vi "PS_Main_two_polarimeters.vi"() -> ()   [LabVIEW 2011]
uses:
  PS_Global.vi
  <vilib>/express/express arith-compare/Formula/XNode/ExpressFormulaBlockNode.xnode
panel:
  out "Offsets at Both Wave Plate Settings":dbl[][](array[numeric])
  in  "Polarimeter Angles":dbl[](array[numeric])
  out "Running Std":dbl[](array[numeric]) format="%#.2g%"
  out "Running Average":dbl[](array[numeric]) format="%#.1f%"
  out "Next Pol Value":dbl[](array[numeric])
  out "Polarization Graph":dynamicdata(graph)
  out "Offset: Laser off":dbl[](array[numeric])
  out "Offset: Laser on":dbl[](array[numeric])
  out "Corrected Lo":dbl[](array[numeric])
  out "Corrected Hi":dbl[](array[numeric])
  out "Optical Polarization":dbl[](array[numeric]) format="%#.1f%"
  out "Nuclear Polarization":dbl[](array[numeric]) format="%#.1f%"
  out "Std Lo":dbl[](array[numeric]) format="%.4f"
  out "Std Hi":dbl[](array[numeric]) format="%.4f"
  out "Mean Lo":dbl[](array[numeric]) format="%.4f"
  out "Mean Hi":dbl[](array[numeric]) format="%.4f"
  in  "# in avg":i32=1000
  in  "Init Running Avg":bool
  out "Counter":i32=1000
  out "Numbers to Avg":dbl[](array[numeric])
  in  "New Discharge ON":bool
  in  "Pressure Calib":dbl=0.553
  out "LCR V Min":dbl
  out "LCR Min V":dbl
  out "LCR Max V":dbl
  out "LCR Calibration Plot":cluster{"Y":dbl[], "Y":dbl[]}[](graph)
  in  "Calibrate LCR":bool
  in  "Discharge Voltage":dbl=10.3
  in  "Cell Pressure":dbl
  in  "stop":bool
  out "Heartbeat":string
  in  "Set All Offsets":bool
  in  "Run Polarimeter?":bool=TRUE
  out "Laser Global":bool
  in  "C8 Line?":bool caption="Laser State"
  out "Status":string
  out "Laser Peaks":cluster{dbl[], dbl[]}[](graph)
  out "Laser Peak Voltage Set":dbl format="%#_g V"
  in  "Run Laser Peak Find":bool
  in  "Lower Voltge Limit":dbl=1.2
  in  "Upper Voltage Limit":dbl=4.0
  in  "CP In?":bool
  in  "Comment Box":string
  in  "Insert Comment":bool
  in  "Plasma On Length":dbl=0.2
  out "Plasma On":dbl
  out "Plasma State":bool caption="Plasma Ball Status"
  out "Shutter Closed":dbl format="%.0f sec"
  in  "Shutter Set":bool=TRUE
  out "Shutter State":bool=TRUE caption="Shutter Status"
  out "Discharge State":bool caption="Discharge Status"
  in  "Discharge Set":bool
  out "Plasma On":timestamp
  out "Shutter Time":timestamp
  out "log":refnum<file>
  out "VI Running":bool
  out "Off Time":timestamp
  out "On Time":timestamp
  out "Decay Running":bool caption="Status"
  out "Start Time":timestamp
  out "Duration":dbl
  in  "Discharge Interval":dbl=30.0
  in  "Discharge Length":dbl=5.0
  in  "Run Decay":bool
  out "Messages":string
  in  "Laser State Set":bool caption="Laser State"
  in  "Get Signal Offset":bool
  in  "High Signal Extend":i32=280
  out "Signals":dynamicdata(graph) caption="Section"
  in  "High Signal Start":i32=400 caption="Begin Sample"
  in  "Low Signal Start":i32=120 caption="Begin Sample"
  in  "Number of Samples":i32=800
  in  "Sample Rate (Hz)":dbl=4000.0
  # "Set Laser State"
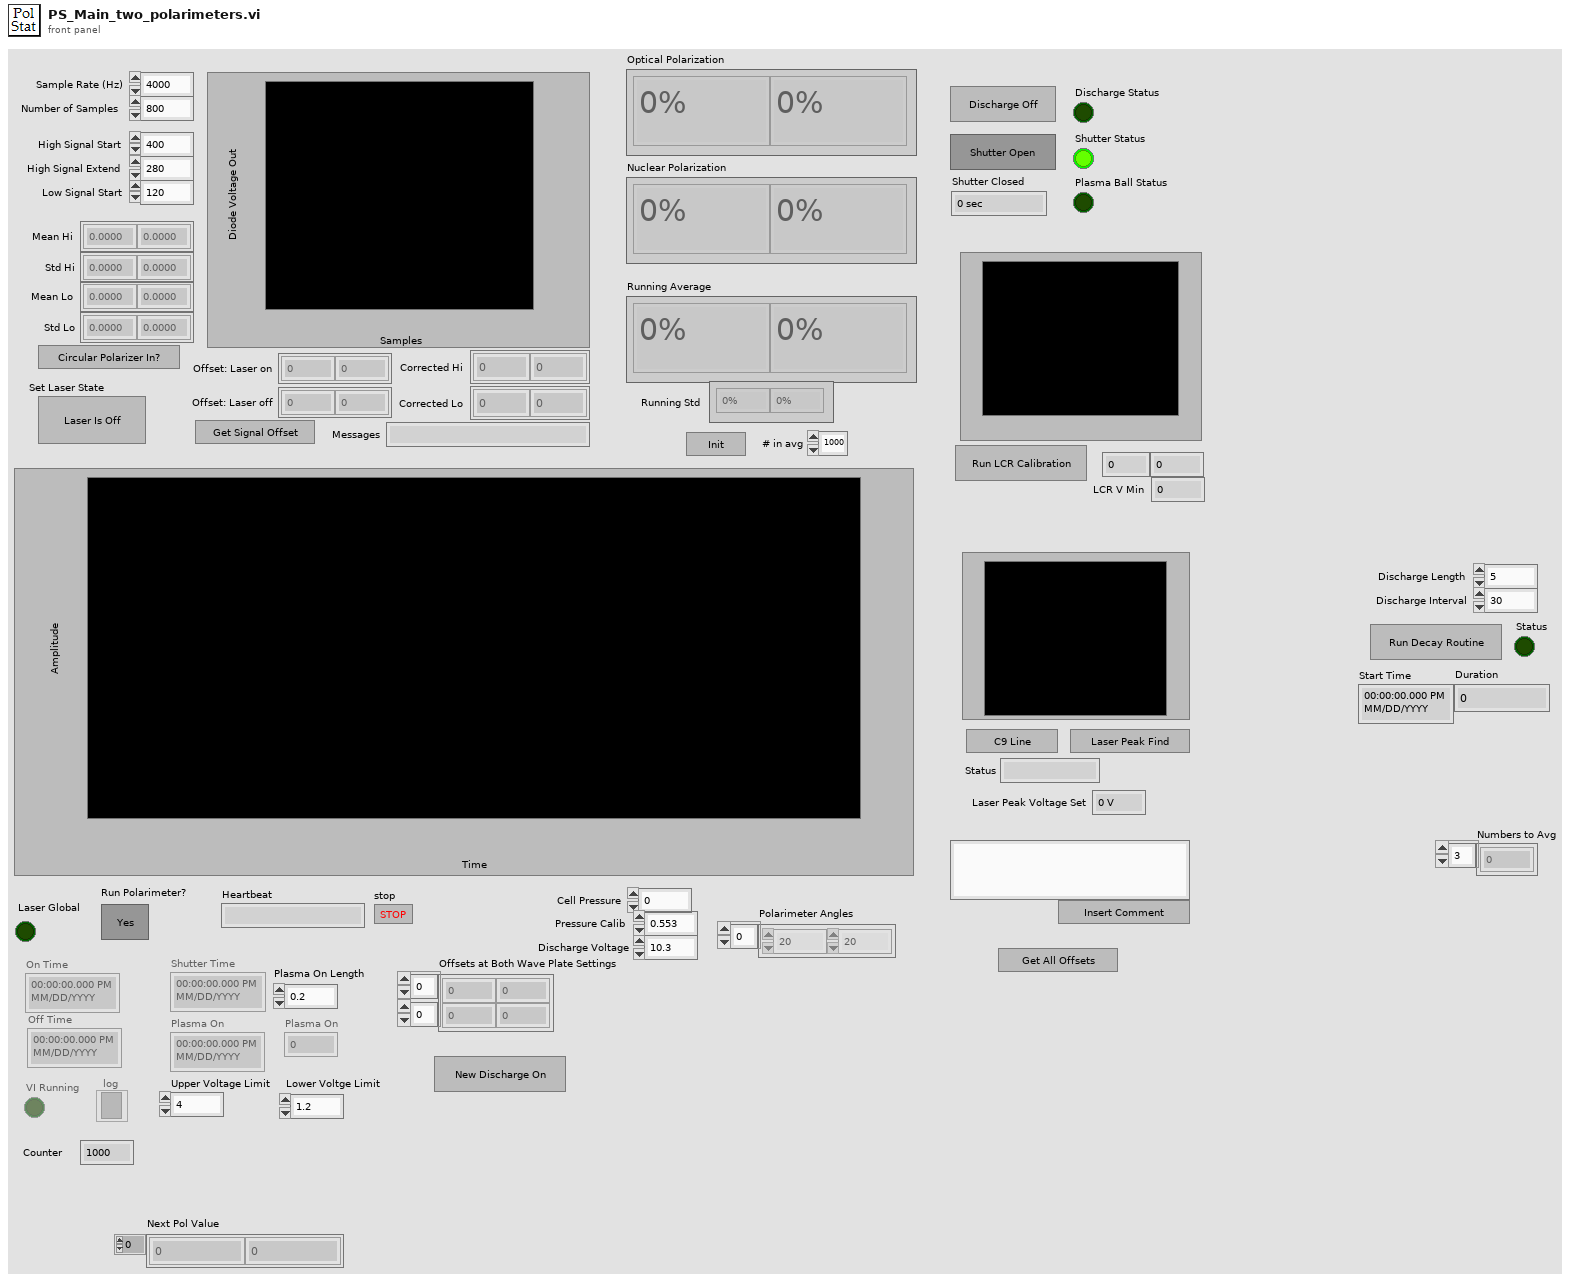
[diagram p1: front panel]
types:
  T1 = enum16{"open", "replace", "create", "open or create", "replace or create", "replace or create with confirmation"}
  T2 = enum8{"Enabled", "Disabled", "Disabled and Grayed Out"}
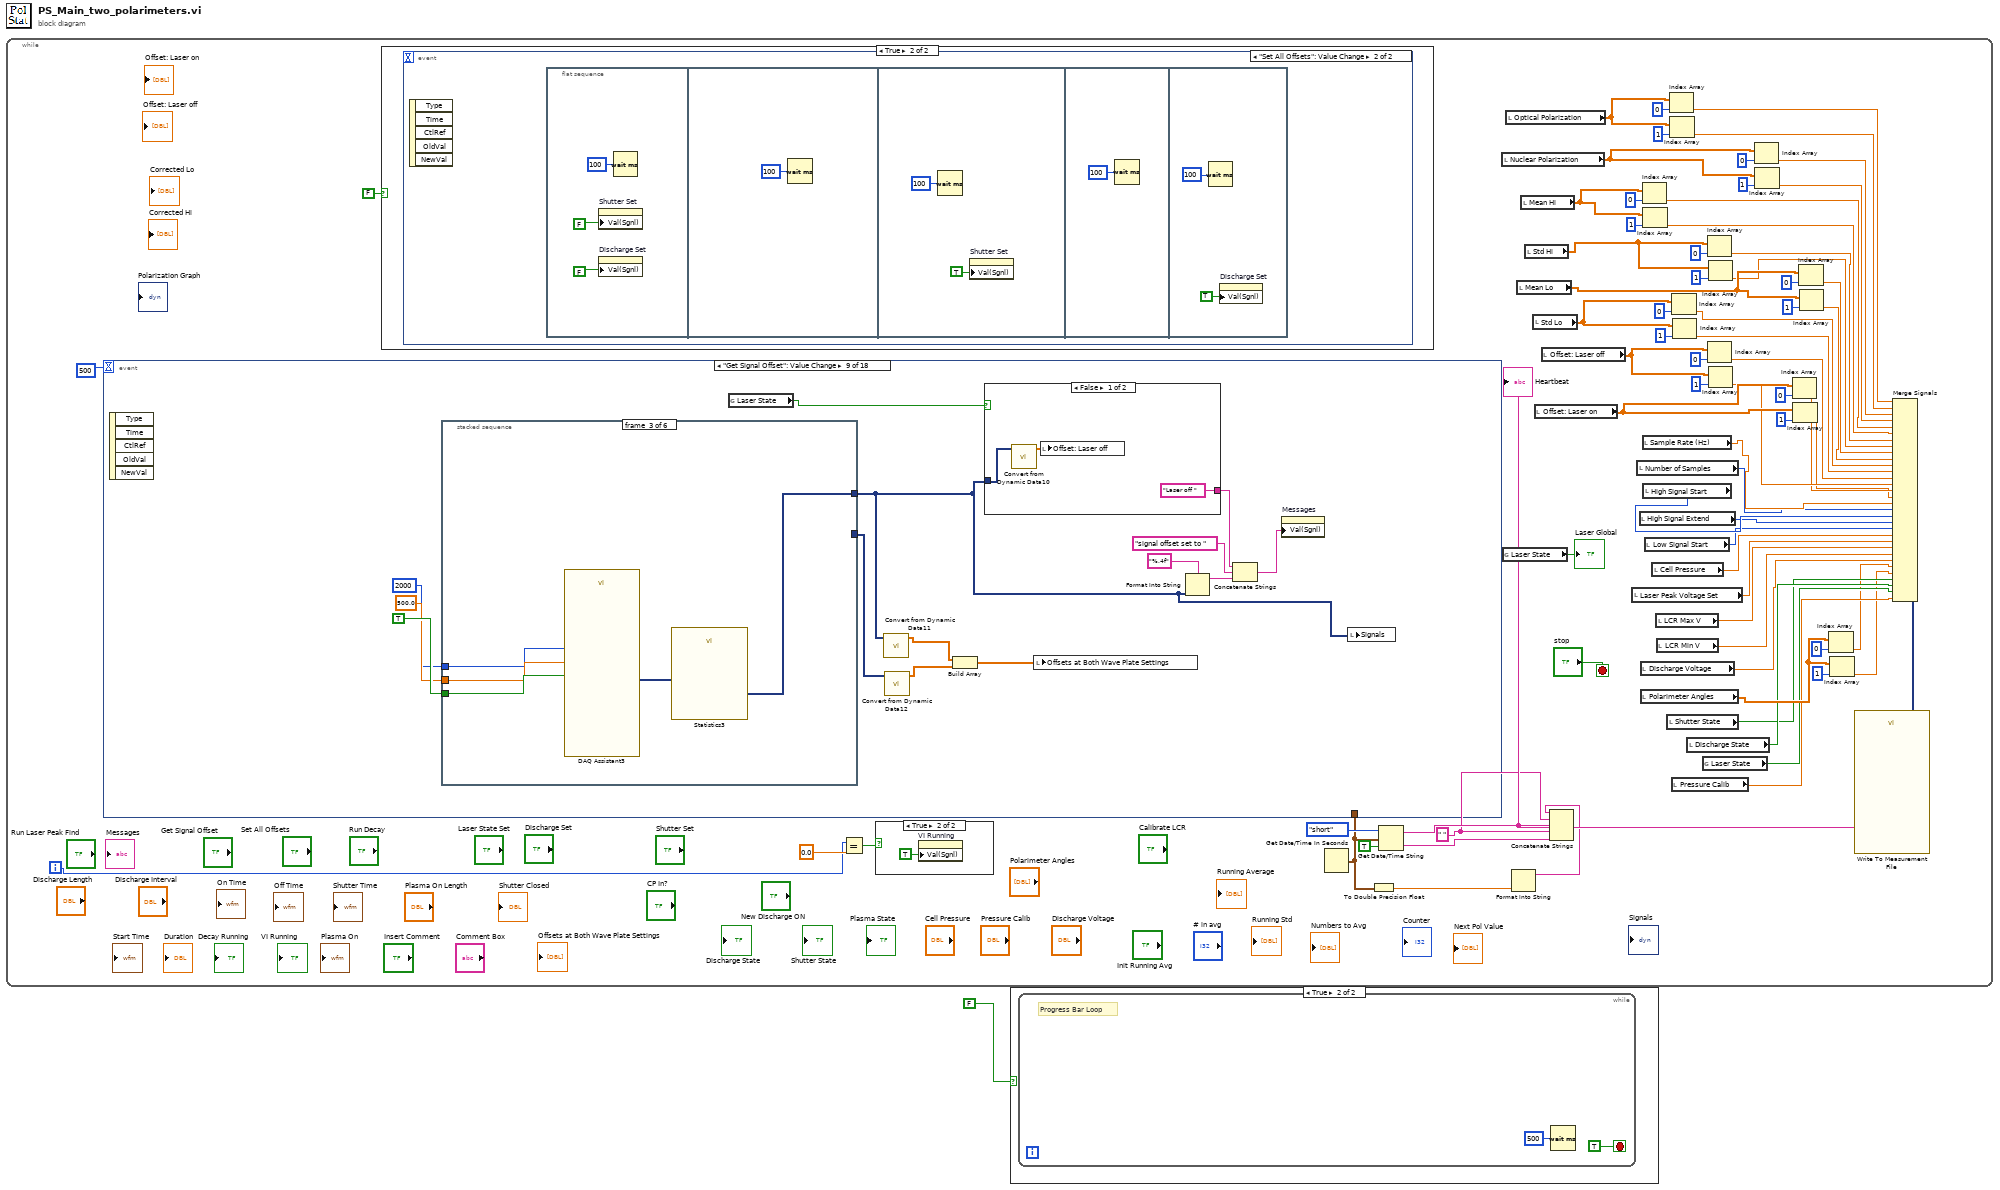
[diagram p0: block diagram]
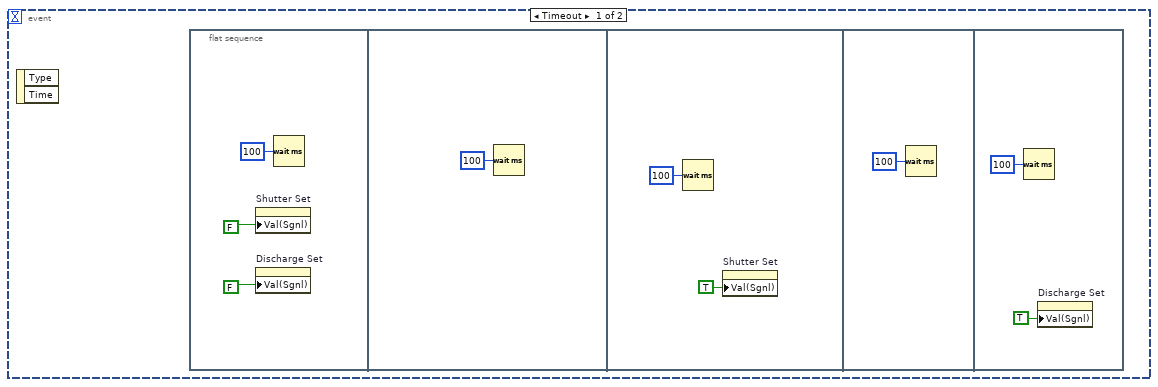
[diagram p4: hidden frame]
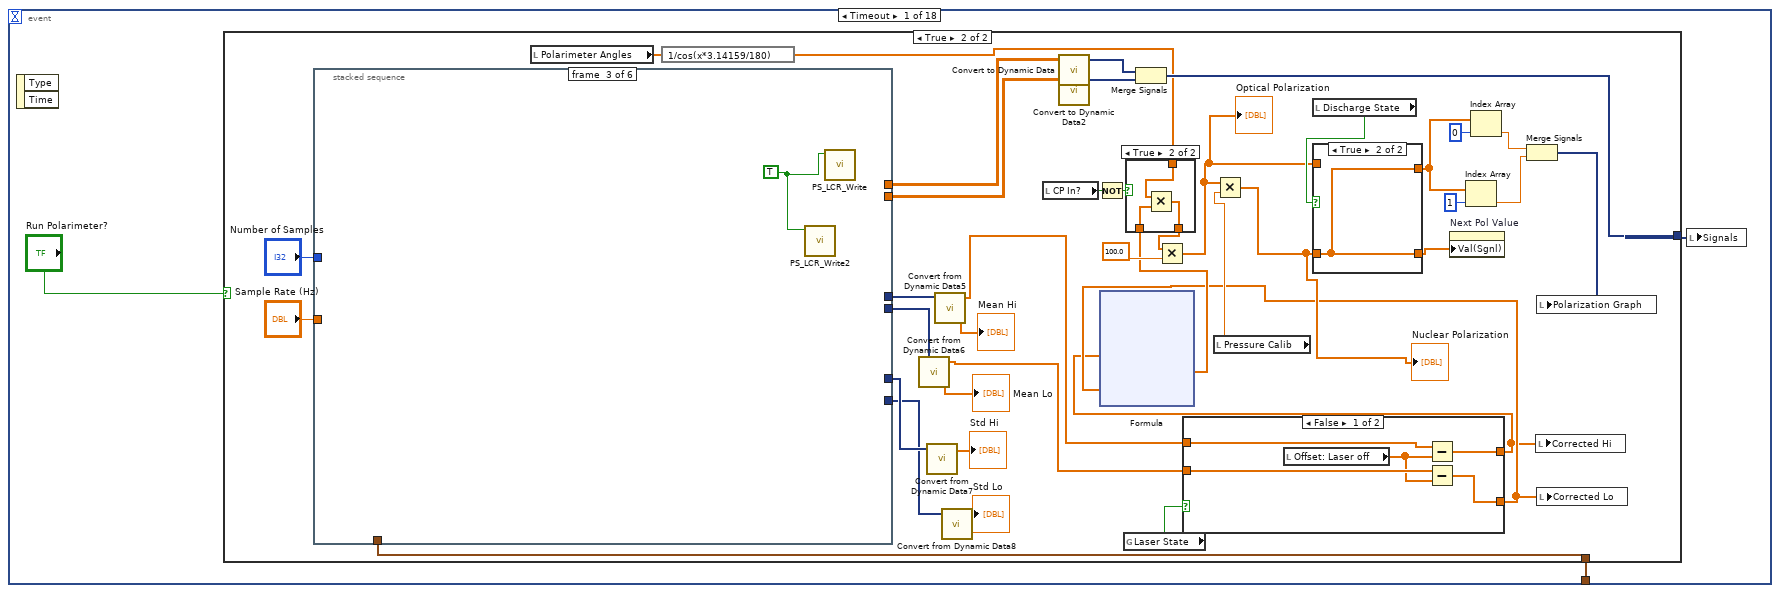
[diagram p6: hidden frame]
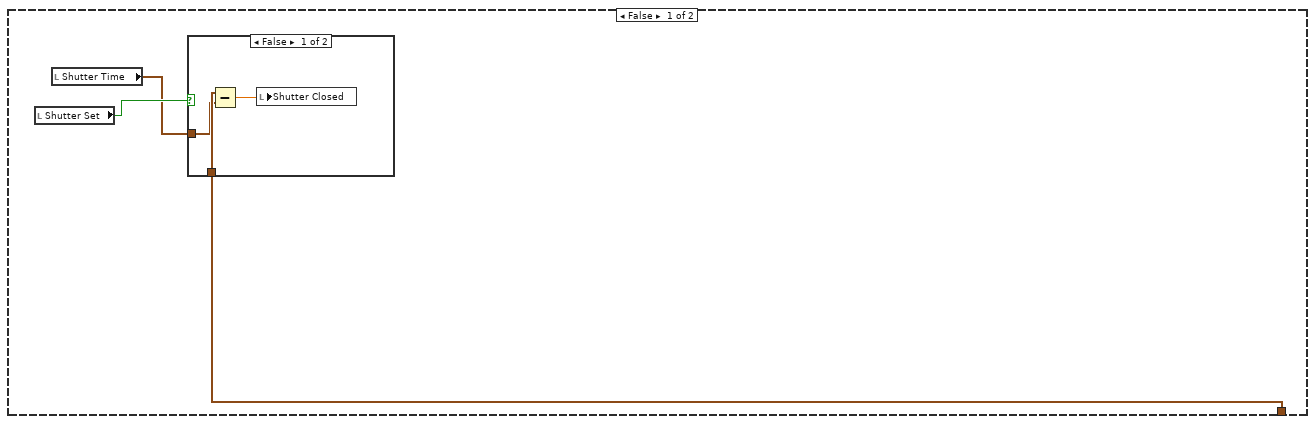
[diagram p7: hidden frame]
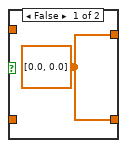
[diagram p9: hidden frame]
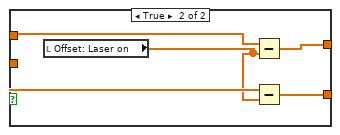
[diagram p11: hidden frame]
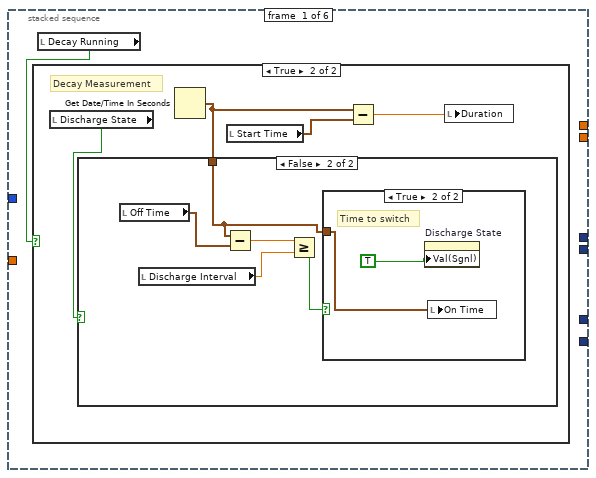
[diagram p12: hidden frame]
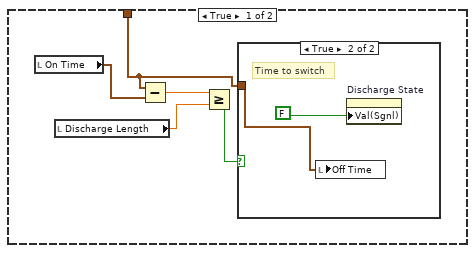
[diagram p14: hidden frame]
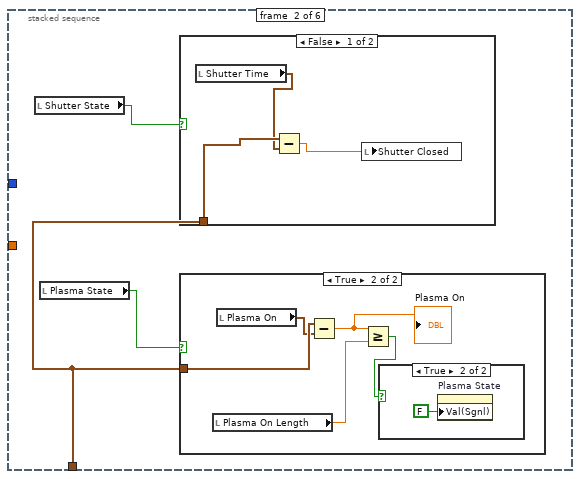
[diagram p17: hidden frame]
diagram:
  n1 = while {
    i -> [w69]
    stop <- "stop" stop-if-true
    w51 = " " ("string")
    n2 = case shown="True" FALSE {
      frame False {
      }
      frame True {
        n3 = event shown="[1] \"Set All Offsets\": Value Change" {
          selector: _ -> [_ _]
          dyn-events: _ -> [_ _]
          timeout: _ -> [_ _]
          event Timeout {
            n4 = event-data() -> ()  [unwired: 1 in, 2 out]
            n5 = flat-sequence {
              frame #0 {
                n6 = property on="Shutter Set" class="Bool (strict)"("Val(Sgnl)"=FALSE ("Value (Signaling)")) -> ()  [unwired: 2 in, 2 out]
                n7 = property on="Discharge Set" class="Bool (strict)"("Val(Sgnl)"=FALSE ("Value (Signaling)")) -> ()  [unwired: 2 in, 2 out]
                n8 = Wait (ms)(milliseconds to wait=u32 100) -> ()  [unwired: 1 out]
              }
              frame #1 {
                n9 = Wait (ms)(milliseconds to wait=u32 100) -> ()  [unwired: 1 out]
              }
              frame #2 {
                n10 = Wait (ms)(milliseconds to wait=u32 100) -> ()  [unwired: 1 out]
                n11 = property on="Shutter Set" class="Bool (strict)"("Val(Sgnl)"=TRUE ("Value (Signaling)")) -> ()  [unwired: 2 in, 2 out]
              }
              frame #3 {
                n12 = Wait (ms)(milliseconds to wait=u32 100) -> ()  [unwired: 1 out]
              }
              frame #4 {
                n13 = Wait (ms)(milliseconds to wait=u32 100) -> ()  [unwired: 1 out]
                n14 = property on="Discharge Set" class="Bool (strict)"("Val(Sgnl)"=TRUE ("Value (Signaling)")) -> ()  [unwired: 2 in, 2 out]
              }
            }
          }
          event "Set All Offsets": Value Change {
            n15 = event-data() -> ()  [unwired: 1 in, 5 out]
            n16 = flat-sequence {
              frame #0 {
                n17 = property on="Shutter Set" class="Bool (strict)"("Val(Sgnl)"=FALSE ("Value (Signaling)")) -> ()  [unwired: 2 in, 2 out]
                n18 = property on="Discharge Set" class="Bool (strict)"("Val(Sgnl)"=FALSE ("Value (Signaling)")) -> ()  [unwired: 2 in, 2 out]
                n19 = Wait (ms)(milliseconds to wait=u32 100) -> ()  [unwired: 1 out]
              }
              frame #1 {
                n20 = Wait (ms)(milliseconds to wait=u32 100) -> ()  [unwired: 1 out]
              }
              frame #2 {
                n21 = Wait (ms)(milliseconds to wait=u32 100) -> ()  [unwired: 1 out]
                n22 = property on="Shutter Set" class="Bool (strict)"("Val(Sgnl)"=TRUE ("Value (Signaling)")) -> ()  [unwired: 2 in, 2 out]
              }
              frame #3 {
                n23 = Wait (ms)(milliseconds to wait=u32 100) -> ()  [unwired: 1 out]
              }
              frame #4 {
                n24 = Wait (ms)(milliseconds to wait=u32 100) -> ()  [unwired: 1 out]
                n25 = property on="Discharge Set" class="Bool (strict)"("Val(Sgnl)"=TRUE ("Value (Signaling)")) -> ()  [unwired: 2 in, 2 out]
              }
            }
          }
        }
      }
    }
    n26 = Equal?(x=w69, y=0.0) -> (x = y?=w71:bool)
    n27 = case shown="True" w71 {
      frame False {
      }
      frame True {
        n28 = property on="VI Running" class="Bool (strict)"("Val(Sgnl)"=TRUE ("Value (Signaling)")) -> ()  [unwired: 2 in, 2 out]
      }
    }
    n29 = Get Date/Time In Seconds() -> (seconds since 1Jan1904=w54:timestamp)
    n30 = event shown="[8] \"Get Signal Offset\": Value Change" {
      selector: _ -> [_ _ _ _ _ _ _ _ _ _ _ _ _ _ _ _ _ _]
      dyn-events: _ -> [_ _ _ _ _ _ _ _ _ _ _ _ _ _ _ _ _ _]
      timeout: 500 -> [_ _ _ _ _ _ _ _ _ _ _ _ _ _ _ _ _ _]
      tunnel: w54 -> [w99 _ _ _ _ _ _ _ _ w309 _ _ _ w353 w359 _ _ _]
      event Timeout {
        n31 = event-data() -> ()  [unwired: 1 in, 2 out]
        n32 = case shown="True" "Run Polarimeter?" {
          tunnel: [_ w136] -> w97
          tunnel: w99 -> [w102 w134]
          frame False {
            n33 = local read "Shutter Set"() -> (w101:bool)
            n34 = local read "Shutter Time"() -> (w100:timestamp)
            n35 = case shown="False" w101 {
              tunnel: w102 -> [w105 _]
              tunnel: w100 -> [w103 _]
              frame False {
                n36 = Subtract(x=w105, y=w103) -> (x-y=w104:dbl)
                n37 = local write "Shutter Closed"(w104) -> ()
              }
              frame True {
              }
            }
          }
          frame True {
            n38 = stacked-sequence {
              tunnel: [_ _ _ w207 _ _] -> w140
              tunnel: "Sample Rate (Hz)" -> [_ _ _ w212 _ w224]
              tunnel: "Number of Samples" -> [_ _ _ w211 _ w216]
              tunnel: [_ _ _ _ _ w220] -> w139
              tunnel: [_ _ _ _ _ w218] -> w125
              tunnel: [_ _ _ w205 _ _] -> w122
              tunnel: [_ _ _ _ _ w217] -> w121
              tunnel: [_ _ _ w204 _ _] -> w120
              tunnel: w134 -> [_ w192 _ _ _ _]
              frame #0 {
                n39 = local read "Decay Running"() -> (w172:bool)
                n40 = case shown="True" w172 {
                  frame False {
                  }
                  frame True {
                    # "Decay Measurement"
                    n41 = local read "Discharge State"() -> (w176:bool)
                    n42 = Get Date/Time In Seconds() -> (seconds since 1Jan1904=w173:timestamp)
                    n43 = case shown="False" w176 {
                      tunnel: w173 -> [w177 w184]
                      frame True {
                        n44 = local read "On Time"() -> (w181:timestamp)
                        n45 = local read "Discharge Length"() -> (w179:dbl)
                        n46 = Subtract(x=w177, y=w181) -> (x-y=w180:dbl)
                        n47 = Greater Or Equal?(x=w180, y=w179) -> (x >= y?=w178:bool)
                        n48 = case shown="True" w178 {
                          tunnel: w177 -> [_ w183]
                          frame False {
                          }
                          frame True {
                            # "Time to switch"
                            n49 = local write "Off Time"(w183) -> ()
                            n50 = property on="Discharge State" class="Bool (strict)"("Val(Sgnl)"=FALSE) -> ()  [unwired: 2 in, 2 out]
                          }
                        }
                      }
                      frame False {
                        n51 = local read "Off Time"() -> (w188:timestamp)
                        n52 = local read "Discharge Interval"() -> (w186:dbl)
                        n53 = Subtract(x=w184, y=w188) -> (x-y=w187:dbl)
                        n54 = Greater Or Equal?(x=w187, y=w186) -> (x >= y?=w185:bool)
                        n55 = case shown="True" w185 {
                          tunnel: w184 -> [_ w190]
                          frame False {
                          }
                          frame True {
                            # "Time to switch"
                            n56 = property on="Discharge State" class="Bool (strict)"("Val(Sgnl)"=TRUE) -> ()  [unwired: 2 in, 2 out]
                            n57 = local write "On Time"(w190) -> ()
                          }
                        }
                      }
                    }
                    n58 = local read "Start Time"() -> (w174:timestamp)
                    n59 = Subtract(x=w173, y=w174) -> (x-y=w175:dbl)
                    n60 = local write "Duration"(w175) -> ()
                  }
                }
              }
              frame #1 {
                n61 = local read "Shutter State"() -> (w191:bool)
                n62 = local read "Plasma State"() -> (w193:bool)
                n63 = case shown="False" w191 {
                  tunnel: w192 -> [w202 _]
                  frame False {
                    n64 = local read "Shutter Time"() -> (w201:timestamp)
                    n65 = Subtract(x=w202, y=w201) -> (x-y=w200:dbl)
                    n66 = local write "Shutter Closed"(w200) -> ()
                  }
                  frame True {
                  }
                }
                n67 = case shown="True" w193 {
                  tunnel: w192 -> [_ w198]
                  frame False {
                  }
                  frame True {
                    n68 = local read "Plasma On Length"() -> (w194:dbl)
                    n69 = local read "Plasma On"() -> (w197:timestamp)
                    n70 = Subtract(x=w198, y=w197) -> (x-y=w196:dbl)
                    "Plasma On" <- w196
                    n71 = Greater Or Equal?(x=w196, y=w194) -> (x >= y?=w195:bool)
                    n72 = case shown="True" w195 {
                      frame False {
                      }
                      frame True {
                        n73 = property on="Plasma State" class="Bool (strict)"("Val(Sgnl)"=FALSE ("Value (Signaling)")) -> ()  [unwired: 2 in, 2 out]
                      }
                    }
                  }
                }
              }
              frame #2 {
                w203 = TRUE ("On/Off")
                n74 = call "PS_LCR_Write2.vi"("On/Off"=w203) -> ()  [unwired: 10 in, 1 out]
                n75 = call "PS_LCR_Write.vi"("On/Off"=w203) -> ()  [unwired: 10 in, 1 out]
              }
              frame #3 {
                n76 = call "DAQ Assistant"("rate"=w212, "number of samples"=w211, "stop (F)"=TRUE) -> ("data"=w210:dynamicdata)  [unwired: 13 in, 3 out]
                n77 = call "Extract Portion of Signal"("Begin Sample"="Low Signal Start", "Signals"=w210) -> ("Section"=w206:dynamicdata)  [unwired: 8 in, 1 out]
                n78 = call "Statistics"("Signals"=w206) -> ("Standard Dev"=w204:dynamicdata, "Arithmetic Mean"=w205:dynamicdata)  [unwired: 24 in, 1 out]
                n79 = call "Convert from Dynamic Data3"("Dynamic Data Type"=w206) -> ("Array"=w207:dbl[][])  [unwired: 3 in]
              }
              frame #4 {
                w213 = FALSE ("On/Off")
                n80 = call "PS_LCR_Write2.vi"("On/Off"=w213) -> ()  [unwired: 10 in, 1 out]
                n81 = call "PS_LCR_Write.vi"("On/Off"=w213) -> ()  [unwired: 10 in, 1 out]
              }
              frame #5 {
                n82 = Add(x=w216, y="High Signal Extend") -> (x+y=w214:i32)
                n83 = call "DAQ Assistant2"("rate"=w224, "number of samples"=w214, "stop (F)"=TRUE) -> ("data"=w223:dynamicdata)  [unwired: 13 in, 3 out]
                n84 = call "Extract Portion of Signal2"("Begin Sample"="High Signal Start", "Signals"=w223) -> ("Section"=w219:dynamicdata)  [unwired: 8 in, 1 out]
                n85 = call "Statistics2"("Signals"=w219) -> ("Standard Dev"=w217:dynamicdata, "Arithmetic Mean"=w218:dynamicdata)  [unwired: 24 in, 1 out]
                n86 = call "Convert from Dynamic Data4"("Dynamic Data Type"=w219) -> ("Array"=w220:dbl[][])  [unwired: 3 in]
              }
            }
            n87 = local read "Polarimeter Angles"() -> (w132:dbl[])
            n88 = expression code="1/cos(x*3.14159/180)"(w132) -> (w131:dbl[])
            n89 = call "Convert from Dynamic Data6"("Dynamic Data Type"=w122) -> ("Array"=w118:dbl[])  [unwired: 3 in]
            "Mean Lo" <- w118
            n90 = call "Convert from Dynamic Data7"("Dynamic Data Type"=w121) -> ("Array"=→"Std Hi":dbl[])  [unwired: 3 in]
            n91 = call "Convert from Dynamic Data5"("Dynamic Data Type"=w125) -> ("Array"=w119:dbl[])  [unwired: 3 in]
            "Mean Hi" <- w119
            n92 = call "Convert from Dynamic Data8"("Dynamic Data Type"=w120) -> ("Array"=→"Std Lo":dbl[])  [unwired: 3 in]
            n93 = local read "CP In?"() -> (w130:bool)
            n94 = call "Convert to Dynamic Data"("2D Array"=w140) -> ("Dynamic Data Type"=w138:dynamicdata)  [unwired: 3 in]
            n95 = call "Convert to Dynamic Data2"("2D Array"=w139) -> ("Dynamic Data Type"=w137:dynamicdata)  [unwired: 3 in]
            n96 = Not(x=w130) -> (.not. x?=w129:bool)
            n97 = global read "PS_Global.vi" "Laser State"() -> (w126:bool)
            n98 = Merge Signals(w138, w137) -> (w136:dynamicdata)
            n99 = case shown="False" w126 {
              tunnel: w118 -> [w164 w168]
              tunnel: w119 -> [w166 w169]
              tunnel: [w165 w171] -> w106
              tunnel: [w163 w170] -> w107
              frame False {
                n100 = local read "Offset: Laser off"() -> (w162:dbl[])
                n101 = Subtract(x=w166, y=w162) -> (x-y=w165:dbl[])
                n102 = Subtract(x=w164, y=w162) -> (x-y=w163:dbl[])
              }
              frame True {
                n103 = local read "Offset: Laser on"() -> (w167:dbl[])
                n104 = Subtract(x=w169, y=w167) -> (x-y=w171:dbl[])
                n105 = Subtract(x=w168, y=w167) -> (x-y=w170:dbl[])
              }
            }
            n106 = xnode "Formula"("X1"=w106, "X2"=w107) -> ("Result"=w117:dbl[])  [unwired: 1 in, 1 out]
            n107 = case shown="True" w129 {
              tunnel: w117 -> [w145 w148]
              tunnel: [w145 w147] -> w133
              tunnel: w131 -> [_ w146]
              frame False {
              }
              frame True {
                n108 = Multiply(x=w146, y=w148) -> (x*y=w147:dbl[])
              }
            }
            n109 = Multiply(x=w133, y=100.0) -> (x*y=w116:dbl[])
            "Optical Polarization" <- w116
            n110 = local read "Pressure Calib"() -> (w127:dbl)
            n111 = Multiply(x=w116, y=w127) -> (x*y=w115:dbl[])
            "Nuclear Polarization" <- w115
            n112 = local read "Discharge State"() -> (w128:bool)
            n113 = case shown="True" w128 {
              tunnel: [w143 w144] -> w112
              tunnel: w116 -> [_ _]
              tunnel: w115 -> [_ w144]
              tunnel: [w143 w144] -> w114
              frame False {
                w143 = dbl[] [0.0, 0.0]
              }
              frame True {
              }
            }
            n114 = property on="Next Pol Value" class="Arr (strict)"("Val(Sgnl)"=w114) -> ()  [unwired: 2 in, 2 out]
            n115 = Index Array(array=w112, index=1) -> (element=w108:dbl)
            n116 = Index Array(array=w112, index=0) -> (element=w109:dbl)
            n117 = Merge Signals(w109, w108) -> (w110:dynamicdata)
            n118 = local write "Corrected Hi"(w106) -> ()
            n119 = local write "Polarization Graph"(w110) -> ()
            n120 = local write "Corrected Lo"(w107) -> ()
          }
        }
        n121 = local write "Signals"(w97) -> ()
      }
      event "Init Running Avg", "Numbers to Avg": Value Change {
        n122 = event-data() -> ()  [unwired: 1 in, 5 out]
        n123 = local read "# in avg"() -> (w228:i32)
        n124 = Initialize Array(0.0 ("element"), w228) -> (w226:dbl[])
        n125 = local write "Counter"(0 ("Counter")) -> ()
        n126 = local write "Numbers to Avg"(w226) -> ()
      }
      event "Next Pol Value": Value Change {
        n127 = event-data() -> ("NewVal"=w230:dbl[])  [unwired: 1 in, 4 out]
        n128 = flat-sequence {
          tunnel: w230 -> [w240]
          tunnel: [w238] -> w229
          tunnel: w229 -> [w242]
          frame #0 {
            n129 = local read "Numbers to Avg"() -> (w239:dbl[])
            n130 = local read "Counter"() -> (w238:i32)
            n131 = local read "# in avg"() -> (w241:i32)
            n132 = Quotient & Remainder(x=w238, y=w241) -> (x-y*floor(x/y)=w237:i32)  [unwired: 1 out]
            n133 = Replace Array Subset(array=w239, new element=w240, index=w237) -> (w236:dbl[])
            n134 = call "Convert to Dynamic Data3"("Array"=w236) -> ("Dynamic Data Type"=w235:dynamicdata)  [unwired: 3 in]
            n135 = call "Statistics4"("Signals"=w235) -> ("Standard Dev"=w233:dynamicdata, "Arithmetic Mean"=w234:dynamicdata)  [unwired: 24 in, 1 out]
            n136 = local write "Numbers to Avg"(w236) -> ()
            n137 = call "Convert from Dynamic Data"("Dynamic Data Type"=w234) -> ("Array"=w232:dbl[])  [unwired: 3 in]
            n138 = local write "Running Average"(w232) -> ()
            n139 = call "Convert from Dynamic Data2"("Channel"=w233) -> ("Array"=w231:dbl[])  [unwired: 3 in]
            n140 = local write "Running Std"(w231) -> ()
          }
          frame #1 {
            n141 = Increment(x=w242) -> (x+1=w243:i32)
            n142 = local write "Counter"(w243) -> ()
          }
        }
      }
      event "New Discharge ON": Value Change {
        n143 = event-data() -> ()  [unwired: 1 in, 5 out]
      }
      event "Cell Pressure": Value Change {
        n144 = event-data() -> ("NewVal"=w249:dbl)  [unwired: 1 in, 4 out]
        n145 = call "PS_Pressure_Cal.vi"("P"=w249) -> ("Pn"=w246:dbl)  [unwired: 9 in, 1 out]
        n146 = local write "Pressure Calib"(w246) -> ()
        n147 = Format Into String(format string="%.2f", w249) -> (resulting string=w252:string)  [unwired: 2 in, 1 out]
        n148 = Format Into String(format string="%.2f", w246) -> (resulting string=w247:string)  [unwired: 2 in, 1 out]
        n149 = Concatenate Strings("Pressure: " ("Messages"), w252, " torr gives " ("string"), w247, "." ("string")) -> (w244:string)
        n150 = property on="Messages" class="Str"("Val(Sgnl)"=w244) -> ()  [unwired: 2 in, 2 out]
      }
      event "Insert Comment": Value Change {
        n151 = event-data() -> ()  [unwired: 1 in, 5 out]
        n152 = local read "Comment Box"() -> (w255:string)
        n153 = local write "Insert Comment"(FALSE ("Insert Comment")) -> ()
        n154 = property on="Messages" class="Str"("Val(Sgnl)"=w255) -> ()  [unwired: 2 in, 2 out]
      }
      event "Calibrate LCR": Value Change {
        n155 = event-data() -> ("NewVal"=w256:bool)  [unwired: 1 in, 4 out]
        n156 = case shown="True" w256 {
          frame False {
          }
          frame True {
            n157 = flat-sequence {
              frame #0 {
                n158 = global write "PS_Global.vi" "Calibration Progress"(u8 0 ("Calibration Progress")) -> ()
                n159 = call "PS_LCR_cal.vi"("Lower Voltge Limit"="Lower Voltge Limit", "Upper Voltage Limit"="Upper Voltage Limit") -> ("Min"=→"LCR V Min":dbl, "XY Graph"=→"LCR Calibration Plot":cluster{"Y":dbl[], "Y":dbl[]}[], "Min Voltage"=→"LCR Min V":dbl, "Max Voltage"=→"LCR Max V":dbl)  [unwired: 6 in]
                n160 = property on="Discharge Set" class="Bool (strict)"("Val(Sgnl)"=TRUE ("Value (Signaling)")) -> ()  [unwired: 2 in, 2 out]
              }
              frame #1 {
                n161 = global write "PS_Global.vi" "Laser Peak Progress"(u8 100 ("Laser Peak Progress")) -> ()
                n162 = property on="Calibrate LCR" class="Bool (strict)"("Val(Sgnl)"=FALSE ("Value (Signaling)")) -> ()  [unwired: 2 in, 2 out]
              }
            }
          }
        }
        n163 = property on="Calibrate LCR" class="Bool (strict)"("Blinking"=w256) -> ()  [unwired: 2 in, 2 out]
      }
      event "Laser State Set": Value Change {
        n164 = event-data() -> ("NewVal"=w268:bool)  [unwired: 1 in, 4 out]
        n165 = local read "Shutter State"() -> (w267:bool)
        n166 = And(x=w267, y=w268) -> (x .and. y?=w269:bool)
        n167 = global write "PS_Global.vi" "Laser State"(w269) -> ()
      }
      event "Get Signal Offset": Value Change {
        n168 = event-data() -> ()  [unwired: 1 in, 5 out]
        n169 = stacked-sequence {
          tunnel: TRUE ("stop (F)") -> [_ _ w290 _ _ w297]
          tunnel: 500.0 ("rate") -> [_ _ w289 _ _ w296]
          tunnel: 2000 ("number of samples") -> [_ _ w288 _ _ w295]
          tunnel: [_ _ w286 _ _ _] -> w274
          tunnel: [_ _ _ _ _ w293] -> w273
          frame #0 {
            w284 = TRUE ("On/Off")
            n170 = call "PS_LCR_Write2.vi"("On/Off"=w284) -> ()  [unwired: 10 in, 1 out]
            n171 = call "PS_LCR_Write.vi"("On/Off"=w284) -> ()  [unwired: 10 in, 1 out]
          }
          frame #1 {
            n172 = Wait (ms)(milliseconds to wait=u32 100) -> ()  [unwired: 1 out]
          }
          frame #2 {
            n173 = call "DAQ Assistant3"("rate"=w289, "number of samples"=w288, "stop (F)"=w290) -> ("data"=w287:dynamicdata)  [unwired: 13 in, 3 out]
            n174 = call "Statistics3"("Signals"=w287) -> ("Arithmetic Mean"=w286:dynamicdata)  [unwired: 24 in, 2 out]
          }
          frame #3 {
            w291 = FALSE ("On/Off")
            n175 = call "PS_LCR_Write2.vi"("On/Off"=w291) -> ()  [unwired: 10 in, 1 out]
            n176 = call "PS_LCR_Write.vi"("On/Off"=w291) -> ()  [unwired: 10 in, 1 out]
          }
          frame #4 {
            n177 = Wait (ms)(milliseconds to wait=u32 100) -> ()  [unwired: 1 out]
          }
          frame #5 {
            n178 = call "DAQ Assistant4"("rate"=w296, "number of samples"=w295, "stop (F)"=w297) -> ("data"=w294:dynamicdata)  [unwired: 13 in, 3 out]
            n179 = call "Statistics5"("Signals"=w294) -> ("Arithmetic Mean"=w293:dynamicdata)  [unwired: 24 in, 2 out]
          }
        }
        n180 = global read "PS_Global.vi" "Laser State"() -> (w275:bool)
        n181 = call "Convert from Dynamic Data11"("Dynamic Data Type"=w274) -> ("Array"=w272:dbl[])  [unwired: 3 in]
        n182 = call "Convert from Dynamic Data12"("Dynamic Data Type"=w273) -> ("Array"=w271:dbl[])  [unwired: 3 in]
        n183 = Build Array(w272, w271) -> (w270:dbl[][])
        n184 = case shown="False" w275 {
          tunnel: w274 -> [w299 w302]
          tunnel: ["Laser off " ("string") "Laser on " ("string")] -> w279
          frame False {
            n185 = call "Convert from Dynamic Data10"("Dynamic Data Type"=w299) -> ("Array"=w298:dbl[])  [unwired: 3 in]
            n186 = local write "Offset: Laser off"(w298) -> ()
          }
          frame True {
            n187 = call "Convert from Dynamic Data9"("Dynamic Data Type"=w302) -> ("Array"=w301:dbl[])  [unwired: 3 in]
            n188 = local write "Offset: Laser on"(w301) -> ()
          }
        }
        n189 = local write "Offsets at Both Wave Plate Settings"(w270) -> ()
        n190 = Format Into String(format string="%.4f", w274) -> (resulting string=w278:string)  [unwired: 2 in, 1 out]
        n191 = Concatenate Strings(w279, "signal offset set to " ("string"), w278) -> (w276:string)
        n192 = property on="Messages" class="Str"("Val(Sgnl)"=w276) -> ()  [unwired: 2 in, 2 out]
        n193 = local write "Signals"(w274) -> ()
      }
      event "Messages": Value Change {
        n194 = event-data() -> ("NewVal"=w308:string)  [unwired: 1 in, 4 out]
        n195 = call <vilib>:"Space Constant.vi"() -> ("String"=w304:string)
        n196 = Get Date/Time String(date format (0)=enum16{"short", "long", "abbreviated"}."short", seconds (now)=w309, want seconds? (F)=TRUE) -> (date string=w312:string, time string=w313:string)
        n197 = local read "log"() -> (w307:refnum<file>)
        n198 = Concatenate Strings(w312, w304, w313, w304, w308, "\r") -> (w306:string)
        n199 = Write to Text File(file (use dialog)=w307, text=w306) -> ()  [unwired: 2 in, 3 out]
      }
      event "VI Running": Value Change {
        w315 = dbl[] [0.0, 0.0] ("Offset: Laser off")
        w318 = "\r"
        w326 = TRUE ("Value (Signaling)")
        w327 = T2."Enabled" ("Disabled")
        # "Runs when VI starts"
        n200 = event-data() -> ()  [unwired: 1 in, 5 out]
        n201 = global read "PS_Global.vi" "Log File"() -> (w330:path)
        n202 = Open/Create/Replace File(file path (use dialog)=w330, operation (0:open)=T1."open or create", access (0:read/write)=enum16{"read/write", "read-only", "write-only"}."write-only") -> (refnum out=w324:refnum<file>)  [unwired: 3 in, 2 out]
        n203 = Set File Position(refnum=w324, from (0:start)=enum16{"start", "end", "current"}."end") -> (refnum out=→"log":refnum<file>)  [unwired: 2 in, 1 out]
        n204 = property on="Discharge Set" class="Bool (strict)"("DisabledEnum"=w327) -> ()  [unwired: 2 in, 2 out]
        n205 = property on="Shutter State" class="Bool (strict)"("Val(Sgnl)"=w326) -> ()  [unwired: 2 in, 2 out]
        n206 = local write "Shutter Set"(w326) -> ()
        n207 = property on="Shutter Set" class="Bool (strict)"("DisabledEnum"=w327) -> ()  [unwired: 2 in, 2 out]
        n208 = global read "PS_Global.vi" "Liquid Crystal Controller Port"() -> (w319:refnum<visa-resource-name>)
        n209 = property on="# in avg" class="DigNum (strict)"("Val(Sgnl)"=10 ("Value (Signaling)")) -> ()  [unwired: 2 in, 2 out]
        n210 = property on="Plasma State" class="Bool (strict)"("Val(Sgnl)"=FALSE ("Value (Signaling)")) -> ()  [unwired: 2 in, 2 out]
        n211 = Concatenate Strings("enable=1" ("write buffer"), w318, "mode=0" ("write buffer"), w318) -> (w321:string)
        n212 = VISA Write(VISA resource name=w319, write buffer=w321) -> ()  [unwired: 1 in, 3 out]
        n213 = local write "Polarimeter Angles"(dbl[] [20.0, 20.0] ("Polarimeter Angles")) -> ()
        n214 = local write "Offset: Laser off"(w315) -> ()
        n215 = local write "Offset: Laser on"(w315) -> ()
      }
      event "Run Laser Peak Find": Value Change {
        n216 = event-data() -> ()  [unwired: 1 in, 5 out]
        n217 = flat-sequence {
          tunnel: [w337] -> w332
          tunnel: ["C8 Line?"] -> w331
          tunnel: w332 -> [w345]
          tunnel: w331 -> [w340]
          frame #0 {
            n218 = global write "PS_Global.vi" "Laser Peak Progress"(u8 0 ("Laser Peak Progress")) -> ()
            n219 = local write "Status"("Running" ("Status")) -> ()
            n220 = property on="Status" class="Str"("Blinking"=TRUE) -> ()  [unwired: 2 in, 2 out]
          }
          frame #1 {
            n221 = call "PS_Laser_Set.vi"("C8 Line?"="C8 Line?") -> ("XY Graph"=→"Laser Peaks":cluster{dbl[], dbl[]}[], "Voltage Set To"=w337:dbl)  [unwired: 8 in]
            "Laser Peak Voltage Set" <- w337
          }
          frame #2 {
            n222 = property on="Status" class="Str"("Blinking"=FALSE) -> ()  [unwired: 2 in, 2 out]
            n223 = local write "Status"("Done!" ("Status")) -> ()
            n224 = case shown="False" w340 {
              tunnel: ["C9 line." ("Messages") "C8 line." ("Messages")] -> w339
              frame False {
              }
              frame True {
              }
            }
            n225 = Format Into String(format string="%.2f", w345) -> (resulting string=w344:string)  [unwired: 2 in, 1 out]
            n226 = Concatenate Strings("Set Laser Peak to " ("Messages"), w344, " V, " ("string"), w339) -> (w341:string)
            n227 = property on="Messages" class="Str"("Val(Sgnl)"=w341) -> ()  [unwired: 2 in, 2 out]
          }
        }
      }
      event "Discharge State": Value Change {
        n228 = event-data() -> ("NewVal"=w351:bool)  [unwired: 1 in, 4 out]
        n229 = call "PS_Discharge_Control.vi"("On/Off"=w351) -> ()  [unwired: 10 in, 1 out]
        n230 = property on="Plasma State" class="Bool (strict)"("Val(Sgnl)"=w351) -> ()  [unwired: 2 in, 2 out]
      }
      event "Plasma State": Value Change {
        n231 = event-data() -> ("NewVal"=w352:bool)  [unwired: 1 in, 4 out]
        n232 = case shown="True" w352 {
          tunnel: w353 -> [_ w354]
          frame False {
          }
          frame True {
            n233 = local write "Plasma On"(w354) -> ()
          }
        }
        n234 = call "PS_Plasma_Ball.vi"("On/Off"=w352) -> ()  [unwired: 10 in, 1 out]
      }
      event "Shutter State": Value Change {
        n235 = event-data() -> ("NewVal"=w357:bool)  [unwired: 1 in, 4 out]
        n236 = local read "Laser State Set"() -> (w356:bool)
        n237 = Not(x=w357) -> (.not. x?=w358:bool)
        n238 = call "PS_Shutter_Control.vi"("On/Off"=w357) -> ()  [unwired: 10 in, 1 out]
        n239 = property on="Shutter Closed" class="DigNum (strict)"("Blinking"=w358) -> ()  [unwired: 2 in, 2 out]
        n240 = And(x=w357, y=w356) -> (x .and. y?=w355:bool)
        n241 = global write "PS_Global.vi" "Laser State"(w355) -> ()
        n242 = case shown="True" w358 {
          tunnel: w359 -> [_ w360]
          frame False {
          }
          frame True {
            n243 = local write "Shutter Time"(w360) -> ()
          }
        }
      }
      event "Run Decay": Value Change {
        n244 = event-data() -> ("NewVal"=w362:bool)  [unwired: 1 in, 4 out]
        n245 = case shown="True" w362 {
          frame False {
            w367 = T2."Enabled" ("Disabled")
            # "Stopping: set discharge and shutter to button state"
            n246 = property on="Discharge Set" class="Bool (strict)"("DisabledEnum"=w367) -> ()  [unwired: 2 in, 2 out]
            n247 = property on="Shutter Set" class="Bool (strict)"("DisabledEnum"=w367) -> ()  [unwired: 2 in, 2 out]
            n248 = local write "Decay Running"(FALSE ("Decay Running")) -> ()
            n249 = local read "Discharge Set"() -> (w369:bool)
            n250 = local read "Shutter Set"() -> (w368:bool)
            n251 = property on="Shutter State" class="Bool (strict)"("Val(Sgnl)"=w368) -> ()  [unwired: 2 in, 2 out]
            n252 = property on="Discharge State" class="Bool (strict)"("Val(Sgnl)"=w369) -> ()  [unwired: 2 in, 2 out]
          }
          frame True {
            w372 = FALSE ("Discharge State")
            w373 = T2."Disabled and Grayed Out" ("Disabled")
            # "Starting: Turn off discharge, close laser shutter"
            n253 = Get Date/Time In Seconds() -> (seconds since 1Jan1904=w371:timestamp)
            n254 = local write "Duration"(0.0 ("Duration")) -> ()
            n255 = local write "Decay Running"(TRUE ("Laser State 2")) -> ()
            n256 = property on="Discharge Set" class="Bool (strict)"("DisabledEnum"=w373) -> ()  [unwired: 2 in, 2 out]
            n257 = property on="Shutter Set" class="Bool (strict)"("DisabledEnum"=w373) -> ()  [unwired: 2 in, 2 out]
            n258 = local write "Start Time"(w371) -> ()
            n259 = property on="Discharge State" class="Bool (strict)"("Val(Sgnl)"=w372) -> ()  [unwired: 2 in, 2 out]
            n260 = property on="Shutter State" class="Bool (strict)"("Val(Sgnl)"=w372) -> ()  [unwired: 2 in, 2 out]
          }
        }
        n261 = case shown="True" w362 {
          tunnel: ["stopped." ("string") "started." ("string")] -> w363
          frame False {
          }
          frame True {
          }
        }
        n262 = Concatenate Strings("Decay routine " ("string"), w363) -> (w361:string)
        n263 = property on="Messages" class="Str"("Val(Sgnl)"=w361) -> ()  [unwired: 2 in, 2 out]
      }
      event "Discharge Set": Value Change {
        n264 = event-data() -> ("NewVal"=w377:bool)  [unwired: 1 in, 4 out]
        n265 = case shown="True" w377 {
          tunnel: ["off." ("string") "on." ("string")] -> w378
          frame False {
          }
          frame True {
          }
        }
        n266 = Concatenate Strings("Discharge turned " ("string"), w378) -> (w376:string)
        n267 = property on="Discharge State" class="Bool (strict)"("Val(Sgnl)"=w377) -> ()  [unwired: 2 in, 2 out]
        n268 = property on="Messages" class="Str"("Val(Sgnl)"=w376) -> ()  [unwired: 2 in, 2 out]
      }
      event "Shutter Set": Value Change {
        n269 = event-data() -> ("NewVal"=w382:bool)  [unwired: 1 in, 4 out]
        n270 = case shown="False" w382 {
          tunnel: ["closed." ("string") "opened." ("string")] -> w384
          frame False {
          }
          frame True {
          }
        }
        n271 = Concatenate Strings("Shutter " ("string"), w384) -> (w383:string)
        n272 = property on="Messages" class="Str"("Val(Sgnl)"=w383) -> ()  [unwired: 2 in, 2 out]
        n273 = property on="Shutter State" class="Bool (strict)"("Val(Sgnl)"=w382) -> ()  [unwired: 2 in, 2 out]
      }
    }
    n274 = To Double Precision Float(number=w54) -> (double precision float=w53:dbl)
    n275 = Get Date/Time String(date format (0)=enum16{"short", "long", "abbreviated"}."short", seconds (now)=w54, want seconds? (F)=TRUE) -> (date string=w74:string, time string=w73:string)
    n276 = local read "Nuclear Polarization"() -> (w31:dbl[])
    n277 = global read "PS_Global.vi" "Laser State"() -> (→"Laser Global":bool)
    n278 = local read "Optical Polarization"() -> (w48:dbl[])
    n279 = Format Into String(w53) -> (resulting string=w52:string)  [unwired: 3 in, 1 out]
    n280 = local read "Mean Lo"() -> (w26:dbl[])
    n281 = local read "Mean Hi"() -> (w28:dbl[])
    n282 = local read "Std Hi"() -> (w27:dbl[])
    n283 = local read "Std Lo"() -> (w25:dbl[])
    n284 = local read "Offset: Laser on"() -> (w23:dbl[])
    n285 = local read "Offset: Laser off"() -> (w24:dbl[])
    n286 = Concatenate Strings(w52, w51, w74, w51, w73) -> (w72:string)
    "Heartbeat" <- w72
    n287 = local read "Laser Peak Voltage Set"() -> (w59:dbl)
    n288 = local read "Number of Samples"() -> (w64:i32)
    n289 = local read "High Signal Extend"() -> (w62:i32)
    n290 = local read "Discharge Voltage"() -> (w56:dbl)
    n291 = local read "Polarimeter Angles"() -> (w8:dbl[])
    n292 = Index Array(array=w28, index=0) -> (element=w22:dbl)
    n293 = local read "Sample Rate (Hz)"() -> (w65:dbl)
    n294 = Index Array(array=w28, index=1) -> (element=w21:dbl)
    n295 = local read "High Signal Start"() -> (w63:i32)
    n296 = local read "Low Signal Start"() -> (w61:i32)
    n297 = local read "Cell Pressure"() -> (w60:dbl)
    n298 = local read "LCR Max V"() -> (w58:dbl)
    n299 = local read "LCR Min V"() -> (w57:dbl)
    n300 = local read "Shutter State"() -> (w4:bool)
    n301 = Index Array(array=w48, index=0) -> (element=w47:dbl)
    n302 = Index Array(array=w48, index=1) -> (element=w46:dbl)
    n303 = Index Array(array=w25, index=0) -> (element=w16:dbl)
    n304 = local read "Pressure Calib"() -> (w7:dbl)
    n305 = Index Array(array=w25, index=1) -> (element=w15:dbl)
    n306 = local read "Discharge State"() -> (w5:bool)
    n307 = global read "PS_Global.vi" "Laser State"() -> (w6:bool)
    n308 = Index Array(array=w27, index=0) -> (element=w20:dbl)
    n309 = Index Array(array=w24, index=0) -> (element=w14:dbl)
    n310 = Index Array(array=w27, index=1) -> (element=w19:dbl)
    n311 = Index Array(array=w24, index=1) -> (element=w13:dbl)
    n312 = Index Array(array=w31, index=0) -> (element=w30:dbl)
    n313 = Index Array(array=w31, index=1) -> (element=w29:dbl)
    n314 = Index Array(array=w23, index=0) -> (element=w12:dbl)
    n315 = Index Array(array=w23, index=1) -> (element=w11:dbl)
    n316 = Index Array(array=w26, index=0) -> (element=w18:dbl)
    n317 = Index Array(array=w26, index=1) -> (element=w17:dbl)
    n318 = Index Array(array=w8, index=0) -> (element=w3:dbl)
    n319 = Index Array(array=w8, index=1) -> (element=w2:dbl)
    n320 = Merge Signals(w47, w46, w30, w29, w22, w21, w20, w19, w18, w17, w16, w15, w14, w13, w12, w11, w65, w64, w63, w62, w61, w60, w59, w58, w57, w56, w3, w2, w4, w5, w6, w7) -> (w55:dynamicdata)
    n321 = call "Write To Measurement File"("Signals"=w55, "Comment"=w72) -> ()  [unwired: 15 in, 3 out]
  }
  n322 = case shown="True" FALSE {
    frame False {
    }
    frame True {
      n323 = while {
        stop <- TRUE stop-if-true
        # "Progress Bar Loop"
        n324 = Wait (ms)(milliseconds to wait=u32 500) -> ()  [unwired: 1 out]
      }
    }
  }
